vi "Lvi Board Serial Number.vi"(8 "error in (no error)":errorcluster, 11 "TaskRef":i32) -> (0 "error out":errorcluster, 1 "function return":i32, 2 "SerialNumber":u32, 3 "TaskRef out":i32)   [LabVIEW 2022 SP3, in "DtLvLink.lvlib"]
doc: "Calls directly into the entry points of the DLL of the Data Acq SDK to return the serial number of the device. This VI is used by the higher-level VI, DtOLGetBoard."
uses:
  DtLvLink.lvlib
  <userlib>/LV-Link3/DtLvLink_64.dll
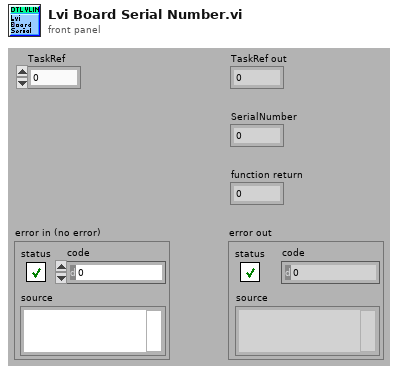
[diagram p1: front panel]
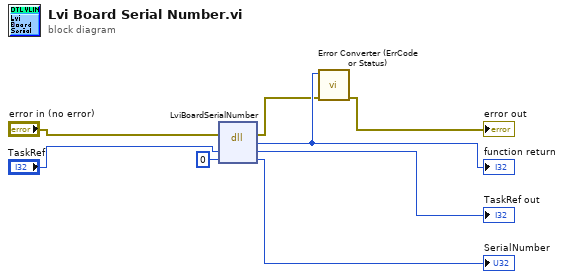
[diagram p0: block diagram]
diagram:
  n1 = dll-call lib="C:/Program Files/National Instruments/LabVIEW 2022/user.lib/LV-Link3/DtLvLink_64.*" fn="LviBoardSerialNumber"(error in="error in (no error)", "TaskRef"="TaskRef", "SerialNumber"=u32 0) -> (error out=w2:errorcluster, "return type"=w8:i32, "TaskRef"=→"TaskRef out":i32, "SerialNumber"=→"SerialNumber":u32)  [unwired: 2 in, 1 out]
  "function return" <- w8
  n2 = call "Error Converter (ErrCode or Status).vi"("error in (no error)"=w2, "error code"=w8) -> ("error out"=→"error out":errorcluster)  [unwired: 9 in]
